vi "Teleop.vi"(0 "Call Context":T10) -> (6 "SubState 3":T4, 8 "SubState 4":T4, 9 "SubState 5":T9, 11 "Loop 3 Data":T5, 13 "Loop 4 Data":T3, 14 "SubState 0":T4=enum."driver control", 15 "Loop 1 Data":T7, 16 "Loop 0 Data":T8, 17 "SubState 1":T4, 18 "Loop 2 Data":T6, 19 "SubState 2":T4)   [LabVIEW 2013]
uses:
  typedefs/subStates.ctl
  <vilib>/Rock Robotics/WPI/DriverStation/WPI_DriverStationDerivedRobotMode.ctl
  typedefs/singleUseSubstate.ctl
  typedefs/Loop Datatypes/Loop 0 Datatype.ctl
  typedefs/Loop Datatypes/Loop 1 Datatype.ctl
  typedefs/Loop Datatypes/Loop 2 Datatype.ctl
  typedefs/Loop Datatypes/Loop 3 Datatype.ctl
  typedefs/Loop Datatypes/Loop 4 Datatype.ctl
  <vilib>/Rock Robotics/WPI/Joystick/WPI_JoystickDevRef.ctl
  <vilib>/Rock Robotics/WPI/Joystick/WPI_JoystickDeviceEnum.ctl
  typedefs/fg_typedef.ctl
  typedefs/vision enable.ctl
  <vilib>/Rock Robotics/WPI/Joystick/WPI_JoystickGetSetRefNum.vi
panel:
  out "JS3":T1
  out "Drive to DC":bool
  out "JS1":T1
  out "JS2":T1
  out "Exit Value":i32=-1
  # "Loop Data and Substates"
  # "Drive Loop"
  # "Shooter Pneumatics Loop"
  # "Pickup/Passing Belts Loop"
  # "Pickup Arm Loop"
  # "Shifter Loop"
  # "Latch Loop"
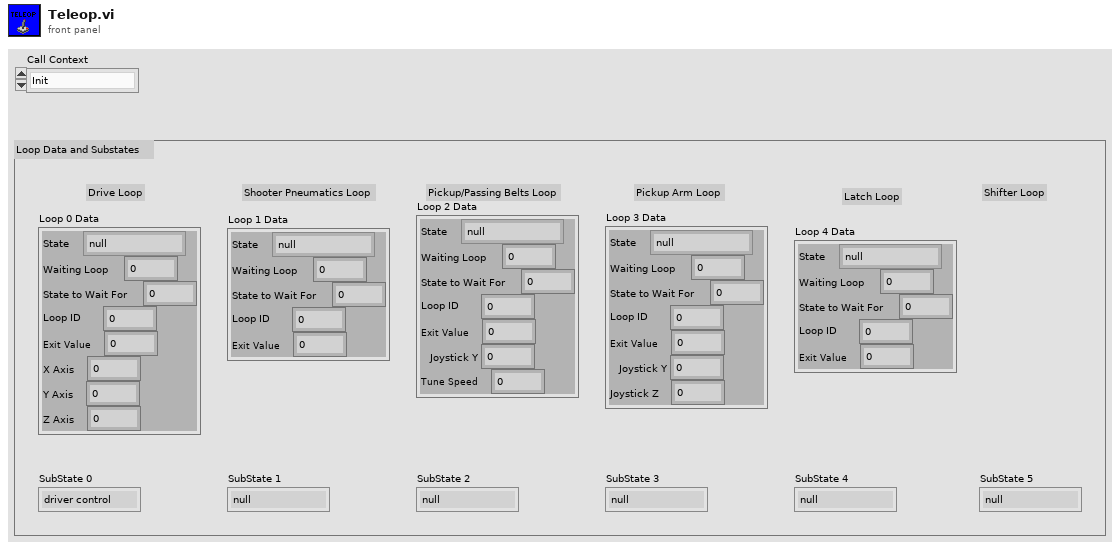
[diagram p1: front panel]
types:
  T1 = typedef "WPI_JoystickDevRef.ctl" = cluster{"Device":T2}
  T2 = typedef "WPI_JoystickDeviceEnum.ctl" = enum16{"USB 1", "USB 2", "USB 3", "USB 4", "Kinect 1", "Kinect 2"}
  T3 = typedef "Loop 4 Datatype.ctl" = cluster{"State":T4, "Waiting Loop":i32, "State to Wait For":i32, "Loop ID":i32, "Exit Value":i32}
  T4 = typedef "subStates.ctl" = enum16{"null", "wait", "driver control", "auto", "manual override", "hold position", "rotate", "pickup", "pass", "load", "goto shoot", "shoot", "end"}
  T5 = typedef "Loop 3 Datatype.ctl" = cluster{"State":T4, "Waiting Loop":i32, "State to Wait For":i32, "Loop ID":i32, "Exit Value":i32, "Joystick Y":dbl, "Joystick Z":dbl}
  T6 = typedef "Loop 2 Datatype.ctl" = cluster{"State":T4, "Waiting Loop":i32, "State to Wait For":i32, "Loop ID":i32, "Exit Value":i32, "Joystick Y":dbl, "Tune Speed":dbl}
  T7 = typedef "Loop 1 Datatype.ctl" = cluster{"State":T4, "Waiting Loop":i32, "State to Wait For":i32, "Loop ID":i32, "Exit Value":i32}
  T8 = typedef "Loop 0 Datatype.ctl" = cluster{"State":T4, "Waiting Loop":i32, "State to Wait For":i32, "Loop ID":i32, "Exit Value":i32, "X Axis":dbl, "Y Axis":dbl, "Z Axis":dbl}
  T9 = typedef "singleUseSubstate.ctl" = enum16{"null", "wait", "shift high", "shift low"}
  T10 = typedef "WPI_DriverStationDerivedRobotMode.ctl" = enum16{"Init", "Execute", "Stop"}
  T11 = cluster{"axis 1 (x)":dbl, "axis 2 (y)":dbl, "axis 3 (throttle)":dbl, "axis 4":dbl, "axis 5":dbl, "axis 6":dbl}
  T12 = typedef "WPI_EncoderDevRef.ctl" = cluster{"DevStatus":errorcluster, "EncoderIndex":T13, "CounterIndex":T14, "DistancePerCount":dbl, "Decoding Type":T15}
  T13 = typedef "FPGA_EncoderIdx.ctl" = enum8{"Enc 0", "Enc 1", "Enc 2", "Enc 3", "Invalid"}
  T14 = typedef "FPGA_CounterCtrSystemIndex.ctl" = enum8{"Ctr 0", "Ctr 1", "Ctr 2", "Ctr 3", "Ctr 4", "Ctr 5", "Ctr 6", "Ctr 7", "Invalid"}
  T15 = typedef "WPI_EncoderType.ctl" = enum16{"1x", "2x", "4x"}
  T16 = typedef "vision enable.ctl" = enum16{"Enable", "Disable", "Stop"}
  T17 = typedef "fg_typedef.ctl" = enum16{"Get", "Set"}
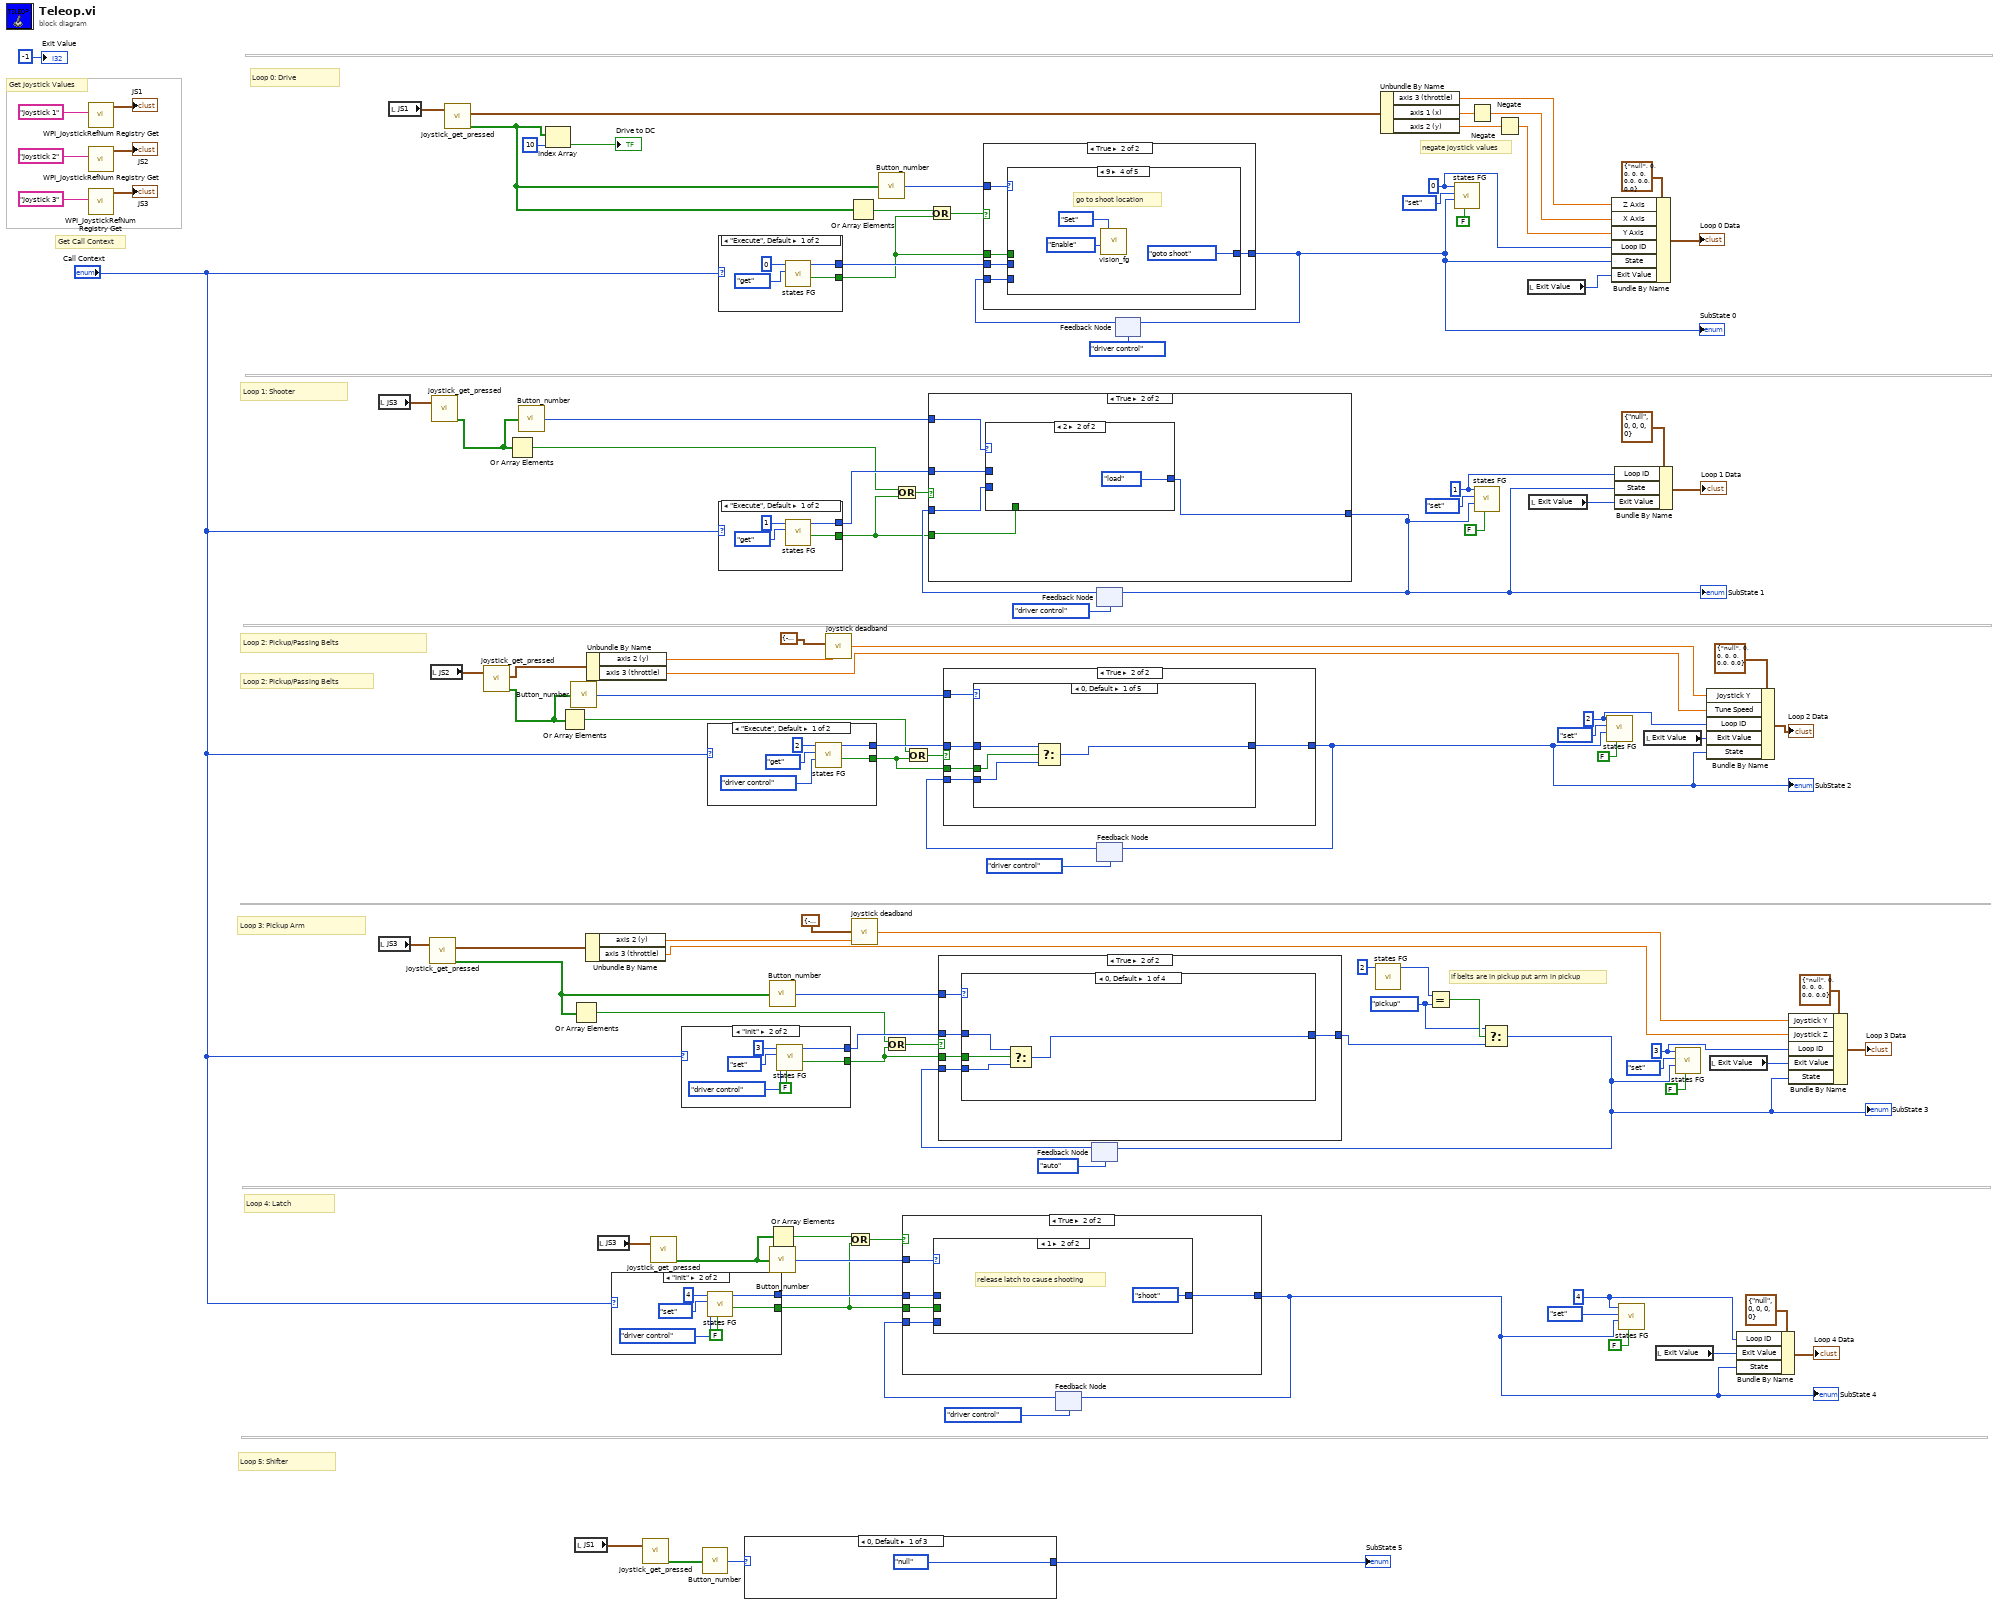
[diagram p0: block diagram]
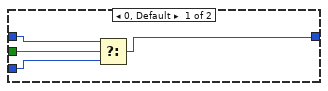
[diagram p3: hidden frame]
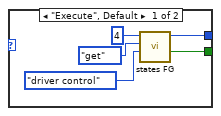
[diagram p4: hidden frame]
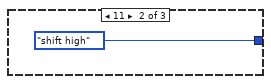
[diagram p5: hidden frame]
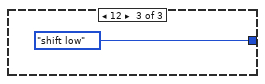
[diagram p6: hidden frame]
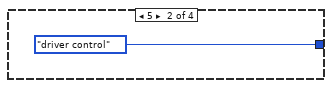
[diagram p8: hidden frame]
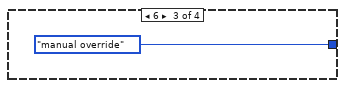
[diagram p9: hidden frame]
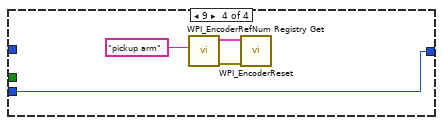
[diagram p10: hidden frame]
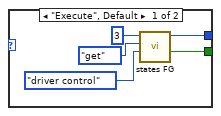
[diagram p11: hidden frame]
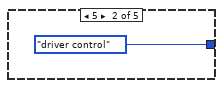
[diagram p13: hidden frame]
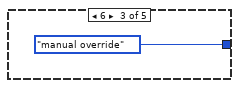
[diagram p14: hidden frame]
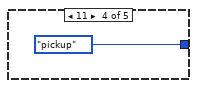
[diagram p15: hidden frame]
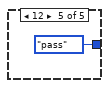
[diagram p16: hidden frame]
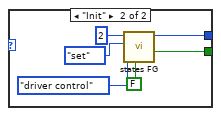
[diagram p17: hidden frame]
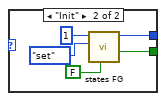
[diagram p18: hidden frame]
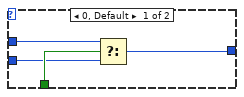
[diagram p20: hidden frame]
diagram:
  w1 = subStates."pickup" ("y")
  w20 = 4 ("Loop ID")
  w87 = 3 ("Loop ID")
  w88 = 2 ("Loop ID")
  w97 = 1 ("Loop ID")
  w99 = 0 ("Loop ID")
  # "if belts are in pickup put arm in pickup"
  # "Loop 2: Pickup/Passing Belts"
  # "negate joystick values"
  # "Get Call Context"
  # "Get Joystick Values"
  # "Loop 4: Latch"
  # "Loop 3: Pickup Arm"
  # "Loop 5: Shifter"
  # "Loop 2: Pickup/Passing Belts"
  # "Loop 1: Shooter"
  # "Loop 0: Drive"
  n1 = call <vilib>:"WPI_JoystickRefNum Registry Get.vi"("refnum name"="Joystick 1") -> ("JoystickDevRef"=→"JS1":T1)  [unwired: 9 in, 1 out]
  n2 = call <vilib>:"WPI_JoystickRefNum Registry Get.vi"("refnum name"="Joystick 2") -> ("JoystickDevRef"=→"JS2":T1)  [unwired: 9 in, 1 out]
  n3 = call <vilib>:"WPI_JoystickRefNum Registry Get.vi"("refnum name"="Joystick 3") -> ("JoystickDevRef"=→"JS3":T1)  [unwired: 9 in, 1 out]
  n4 = local read "JS3"() -> (w64:T1)
  n5 = local read "JS3"() -> (w49:T1)
  n6 = local read "JS1"() -> (w65:T1)
  n7 = call "joystick_get_pressed.vi"("JoystickDevRef 2"=w49) -> ("Axes"=w53:T11, "Buttons Pressed?"=w29:bool[])  [unwired: 1 in, 2 out]
  n8 = local read "JS2"() -> (w36:T1)
  n9 = call "joystick_get_pressed.vi"("JoystickDevRef 2"=w64) -> ("Buttons Pressed?"=w31:bool[])  [unwired: 1 in, 3 out]
  n10 = call "joystick_get_pressed.vi"("JoystickDevRef 2"=w65) -> ("Axes"=w69:T11, "Buttons Pressed?"=w44:bool[])  [unwired: 1 in, 2 out]
  n11 = call "joystick_get_pressed.vi"("JoystickDevRef 2"=w36) -> ("Axes"=w17:T11, "Buttons Pressed?"=w18:bool[])  [unwired: 1 in, 2 out]
  n12 = Or Array Elements(Boolean array=w31) -> (logical OR=w56:bool)
  n13 = call "Button_number.vi"("Button Array"=w31) -> ("Button Pressed"=w58:i32)
  n14 = Index Array(array=w44, index=10) -> (element=→"Drive to DC":bool)
  n15 = Or Array Elements(Boolean array=w18) -> (logical OR=w35:bool)
  n16 = call "Button_number.vi"("Button Array"=w18) -> ("Button Pressed"=w34:i32)
  n17 = Or Array Elements(Boolean array=w29) -> (logical OR=w52:bool)
  n18 = local read "JS1"() -> (w39:T1)
  n19 = Unbundle By Name(w53) -> ("axis 2 (y)"=w47:dbl, "axis 3 (throttle)"=w13:dbl)
  n20 = Unbundle By Name(w17) -> ("axis 2 (y)"=w28:dbl, "axis 3 (throttle)"=w15:dbl)
  n21 = local read "JS3"() -> (w12:T1)
  n22 = case shown="\"Init\"" "Call Context" {
    tunnel: [w118 w124] -> w7
    tunnel: [w116 w121] -> w22
    frame "Execute", Default {
      n23 = call "states FG.vi"("subState in"=subStates."driver control", "menu (get)"=enum16{"set", "get"}."get", "Loop ID"=4) -> ("exit out"=w118:bool, "subState out"=w116:T4)  [unwired: 5 in, 2 out]
    }
    frame "Init" {
      n24 = call "states FG.vi"("exit in"=FALSE, "subState in"=subStates."driver control", "menu (get)"=enum16{"set", "get"}."set", "Loop ID"=4) -> ("exit out"=w124:bool, "subState out"=w121:T4)  [unwired: 4 in, 2 out]
    }
  }
  n25 = call "joystick_get_pressed.vi"("JoystickDevRef 2"=w39) -> ("Buttons Pressed?"=w41:bool[])  [unwired: 1 in, 3 out]
  n26 = call "joystick_get_pressed.vi"("JoystickDevRef 2"=w12) -> ("Buttons Pressed?"=w11:bool[])  [unwired: 1 in, 3 out]
  n27 = case shown="\"Init\"" "Call Context" {
    tunnel: [w129 w135] -> w50
    tunnel: [w127 w132] -> w85
    frame "Execute", Default {
      n28 = call "states FG.vi"("subState in"=subStates."driver control", "menu (get)"=enum16{"set", "get"}."get", "Loop ID"=3) -> ("exit out"=w129:bool, "subState out"=w127:T4)  [unwired: 5 in, 2 out]
    }
    frame "Init" {
      n29 = call "states FG.vi"("exit in"=FALSE, "subState in"=subStates."driver control", "menu (get)"=enum16{"set", "get"}."set", "Loop ID"=3) -> ("exit out"=w135:bool, "subState out"=w132:T4)  [unwired: 4 in, 2 out]
    }
  }
  n30 = call "Button_number.vi"("Button Array"=w41) -> ("Button Pressed"=w40:i32)
  n31 = case shown="\"Execute\", Default" "Call Context" {
    tunnel: [w140 w146] -> w55
    tunnel: [w138 w143] -> w104
    frame "Execute", Default {
      n32 = call "states FG.vi"("subState in"=subStates."driver control", "menu (get)"=enum16{"set", "get"}."get", "Loop ID"=2) -> ("exit out"=w140:bool, "subState out"=w138:T4)  [unwired: 5 in, 2 out]
    }
    frame "Init" {
      n33 = call "states FG.vi"("exit in"=FALSE, "subState in"=subStates."driver control", "menu (get)"=enum16{"set", "get"}."set", "Loop ID"=2) -> ("exit out"=w146:bool, "subState out"=w143:T4)  [unwired: 4 in, 2 out]
    }
  }
  n34 = case shown="\"Execute\", Default" "Call Context" {
    tunnel: [w150 w155] -> w62
    tunnel: [w149 w153] -> w102
    frame "Execute", Default {
      n35 = call "states FG.vi"("menu (get)"=enum16{"set", "get"}."get", "Loop ID"=0) -> ("exit out"=w150:bool, "subState out"=w149:T4)  [unwired: 6 in, 2 out]
    }
    frame "Init" {
      n36 = call "states FG.vi"("exit in"=FALSE, "menu (get)"=enum16{"set", "get"}."set", "Loop ID"=0) -> ("exit out"=w155:bool, "subState out"=w153:T4)  [unwired: 5 in, 2 out]
    }
  }
  n37 = case shown="\"Execute\", Default" "Call Context" {
    tunnel: [w159 w164] -> w59
    tunnel: [w158 w162] -> w101
    frame "Execute", Default {
      n38 = call "states FG.vi"("menu (get)"=enum16{"set", "get"}."get", "Loop ID"=1) -> ("exit out"=w159:bool, "subState out"=w158:T4)  [unwired: 6 in, 2 out]
    }
    frame "Init" {
      n39 = call "states FG.vi"("exit in"=FALSE, "menu (get)"=enum16{"set", "get"}."set", "Loop ID"=1) -> ("exit out"=w164:bool, "subState out"=w162:T4)  [unwired: 5 in, 2 out]
    }
  }
  n40 = case shown="0, Default" w40 {
    tunnel: [singleUseSubstate."null" ("Enum") singleUseSubstate."shift high" ("Enum") singleUseSubstate."shift low" ("Enum")] -> w77
    frame 0, Default {
    }
    frame 11 {
    }
    frame 12 {
    }
  }
  "SubState 5" <- w77
  n41 = call "Button_number.vi"("Button Array"=w29) -> ("Button Pressed"=w51:i32)
  n42 = call "Button_number.vi"("Button Array"=w11) -> ("Button Pressed"=w8:i32)
  n43 = Or Array Elements(Boolean array=w11) -> (logical OR=w10:bool)
  n44 = call "joystick deadband.vi"("Joystick In"=w28, "Deadband Range"=cluster{"Deadband Min":dbl, "Deadband Max":dbl} {"Deadband Min"=-0.05, "Deadband Max"=0.05}) -> ("Joystick Out"=w16:dbl)  [unwired: 4 in]
  n45 = Or(x=w10, y=w7) -> (x .or. y?=w9:bool)
  n46 = Or Array Elements(Boolean array=w44) -> (logical OR=w63:bool)
  n47 = call "joystick deadband.vi"("Joystick In"=w47, "Deadband Range"=cluster{"Deadband Min":dbl, "Deadband Max":dbl} {"Deadband Min"=-0.05, "Deadband Max"=0.05}) -> ("Joystick Out"=w14:dbl)  [unwired: 4 in]
  n48 = call "Button_number.vi"("Button Array"=w44) -> ("Button Pressed"=w68:i32)
  n49 = Or(x=w52, y=w50) -> (x .or. y?=w54:bool)
  n50 = Or(x=w56, y=w59) -> (x .or. y?=w60:bool)
  n51 = Or(x=w35, y=w55) -> (x .or. y?=w57:bool)
  n52 = Or(x=w63, y=w62) -> (x .or. y?=w61:bool)
  n53 = feedback #1(subStates."driver control" ("Drive SubState")) -> (w25:T4)
  n54 = case shown="True" w9 {
    tunnel: w25 -> [w170 w172]
    tunnel: [w170 w171] -> w48
    tunnel: w22 -> [_ w174]
    tunnel: w8 -> [_ w175]
    tunnel: w7 -> [_ w173]
    frame False {
      # "*yawn* nothing to do...wire through the previous state"
    }
    frame True {
      n55 = case shown="1" w175 {
        tunnel: w174 -> [w178 _]
        tunnel: w173 -> [w179 _]
        tunnel: w172 -> [w177 _]
        tunnel: [w176 subStates."shoot" ("Drive SubState")] -> w171
        frame 0, Default {
          n56 = Select(t=w178, s=w179, f=w177) -> (s? t:f=w176:T4)
        }
        frame 1 {
          # "release latch to cause shooting"
        }
      }
    }
  }
  "SubState 4" <- w48
  n57 = feedback-in #1(w48) -> ()
  n58 = feedback #2(subStates."auto" ("Drive SubState")) -> (w82:T4)
  n59 = case shown="True" w54 {
    tunnel: w82 -> [w181 w182]
    tunnel: [w181 w183] -> w4
    tunnel: w85 -> [_ w184]
    tunnel: w51 -> [_ w186]
    tunnel: w50 -> [_ w185]
    frame False {
      # "boring drivers, not pressing anything...wire through the previous state"
    }
    frame True {
      n60 = case shown="0, Default" w186 {
        tunnel: w185 -> [w190 _ _ _]
        tunnel: w182 -> [w189 _ _ w196]
        tunnel: w184 -> [w188 _ _ _]
        tunnel: [w187 subStates."driver control" ("Drive SubState") subStates."manual override" ("Drive SubState") w196] -> w183
        frame 0, Default {
          n61 = Select(t=w188, s=w190, f=w189) -> (s? t:f=w187:T4)
        }
        frame 5 {
        }
        frame 6 {
        }
        frame 9 {
          n62 = call <vilib>:"WPI_EncoderRefNum Registry Get.vi"("refnum name"="pickup arm") -> ("error out"=w194:errorcluster, "EncoderDevRef"=w193:T12)  [unwired: 9 in]
          n63 = call <vilib>:"WPI_EncoderReset.vi"("error in (no error)"=w194, "EncoderDevRef"=w193) -> ()  [unwired: 8 in, 2 out]
        }
      }
    }
  }
  n64 = feedback #3(subStates."driver control" ("Drive SubState")) -> (w103:T4)
  n65 = case shown="True" w60 {
    tunnel: w103 -> [w197 w201]
    tunnel: [w197 w198] -> w70
    tunnel: w101 -> [_ w202]
    tunnel: w58 -> [_ w200]
    tunnel: w59 -> [_ w199]
    frame False {
      # "nothing pressed here, move along (wire through the previous state)"
    }
    frame True {
      n66 = case shown="2" w200 {
        tunnel: w202 -> [w205 _]
        tunnel: w201 -> [w204 _]
        tunnel: [w203 subStates."load" ("Drive SubState")] -> w198
        tunnel: w199 -> [w206 _]
        frame 0, Default {
          n67 = Select(t=w205, s=w206, f=w204) -> (s? t:f=w203:T4)
        }
        frame 2 {
        }
      }
    }
  }
  "SubState 1" <- w70
  n68 = feedback-in #3(w70) -> ()
  n69 = feedback #4(subStates."driver control" ("Drive SubState")) -> (w107:T4)
  n70 = case shown="True" w57 {
    tunnel: w107 -> [w208 w210]
    tunnel: [w208 w209] -> w27
    tunnel: w104 -> [_ w211]
    tunnel: w34 -> [_ w213]
    tunnel: w55 -> [_ w212]
    frame False {
      # "nothing pressed here, move along obviously and wire through the previous state"
    }
    frame True {
      n71 = case shown="0, Default" w213 {
        tunnel: w212 -> [w217 _ _ _ _]
        tunnel: w211 -> [w216 _ _ _ _]
        tunnel: w210 -> [w215 _ _ _ _]
        tunnel: [w214 subStates."driver control" ("Drive SubState") subStates."manual override" ("Drive SubState") subStates."pickup" ("Drive SubState") subStates."pass" ("Drive SubState")] -> w209
        frame 0, Default {
          n72 = Select(t=w216, s=w217, f=w215) -> (s? t:f=w214:T4)
        }
        frame 5 {
        }
        frame 6 {
        }
        frame 11 {
        }
        frame 12 {
        }
      }
    }
  }
  "SubState 2" <- w27
  n73 = feedback-in #4(w27) -> ()
  n74 = feedback #5(subStates."driver control" ("Drive SubState")) -> (w109:T4)
  n75 = case shown="True" w61 {
    tunnel: w109 -> [w222 w224]
    tunnel: [w222 w223] -> w38
    tunnel: w102 -> [_ w225]
    tunnel: w68 -> [_ w227]
    tunnel: w62 -> [_ w226]
    frame False {
      # "keep current state, no change necessary"
    }
    frame True {
      n76 = case shown="9" w227 {
        tunnel: w226 -> [w231 _ _ _ _]
        tunnel: w225 -> [w230 _ _ _ _]
        tunnel: w224 -> [w229 _ w235 _ w250]
        tunnel: [w228 subStates."driver control" ("Drive SubState") w235 subStates."goto shoot" ("Drive SubState") w246] -> w223
        frame 0, Default {
          n77 = Select(t=w230, s=w231, f=w229) -> (s? t:f=w228:T4)
        }
        frame 7 {
          # "put robot drive in driver control"
          n78 = call "vision_fg.vi"("Action"=vision_enable."Disable", "Menu"=fg_typedef."Set") -> ()  [unwired: 1 in, 2 out]
        }
        frame 8 {
          w238 = vision_enable."Enable" ("y")
          # "toggle vision"
          n79 = call "vision_fg.vi"("Menu"=fg_typedef."Get") -> ("State Out"=w240:T16)  [unwired: 2 in, 1 out]
          n80 = Equal?(x=w240, y=w238) -> (x = y?=w239:bool)
          n81 = Select(t=vision_enable."Disable" ("y"), s=w239, f=w238) -> (s? t:f=w236:T16)
          n82 = call "vision_fg.vi"("Action"=w236, "Menu"=fg_typedef."Set") -> ()  [unwired: 1 in, 2 out]
        }
        frame 9 {
          # "go to shoot location"
          n83 = call "vision_fg.vi"("Action"=vision_enable."Enable", "Menu"=fg_typedef."Set") -> ()  [unwired: 1 in, 2 out]
        }
        frame 10 {
          w247 = subStates."hold position" ("x")
          # "button 10, hold position toggle"
          n84 = Equal?(x=w247, y=w250) -> (x = y?=w249:bool)
          n85 = Select(t=subStates."driver control" ("Drive SubState"), s=w249, f=w247) -> (s? t:f=w246:T4)
        }
      }
    }
  }
  "SubState 0" <- w38
  n86 = feedback-in #5(w38) -> ()
  n87 = call "states FG.vi"("Loop ID"=2) -> ("subState out"=w5:T4)  [unwired: 7 in, 3 out]
  n88 = Unbundle By Name(w69) -> ("axis 3 (throttle)"=w45:dbl, "axis 1 (x)"=w74:dbl, "axis 2 (y)"=w73:dbl)
  n89 = Equal?(x=w5, y=w1) -> (x = y?=w2:bool)
  n90 = call "states FG.vi"("exit in"=FALSE, "subState in"=w38, "menu (get)"=enum16{"set", "get"}."set", "Loop ID"=w99) -> ()  [unwired: 4 in, 4 out]
  n91 = Negate(x=w74) -> (-x=w72:dbl)
  n92 = call "states FG.vi"("exit in"=FALSE, "subState in"=w70, "menu (get)"=enum16{"set", "get"}."set", "Loop ID"=w97) -> ()  [unwired: 4 in, 4 out]
  n93 = Select(t=w1, s=w2, f=w4) -> (s? t:f=w3:T4)
  "SubState 3" <- w3
  n94 = feedback-in #2(w3) -> ()
  n95 = Negate(x=w73) -> (-x=w71:dbl)
  n96 = local read "Exit Value"() -> (w95:i32)
  n97 = local read "Exit Value"() -> (w94:i32)
  n98 = call "states FG.vi"("exit in"=FALSE, "subState in"=w27, "menu (get)"=enum16{"set", "get"}."set", "Loop ID"=w88) -> ()  [unwired: 4 in, 4 out]
  n99 = Bundle By Name(cluster=T8 {"State"=enum."null", "Waiting Loop"=0, "State to Wait For"=0, "Loop ID"=0, "Exit Value"=0, "X Axis"=0.0, "Y Axis"=0.0, "Z Axis"=0.0} ("Cluster"), "Z Axis"=w45, "X Axis"=w72, "Y Axis"=w71, "Loop ID"=w99, "State"=w38, "Exit Value"=w95) -> (→"Loop 0 Data":T8)
  n100 = Bundle By Name(cluster=T7 {"State"=enum."null", "Waiting Loop"=0, "State to Wait For"=0, "Loop ID"=0, "Exit Value"=0} ("Cluster"), "Loop ID"=w97, "State"=w70, "Exit Value"=w94) -> (→"Loop 1 Data":T7)
  n101 = call "states FG.vi"("exit in"=FALSE, "subState in"=w48, "menu (get)"=enum16{"set", "get"}."set", "Loop ID"=w20) -> ()  [unwired: 4 in, 4 out]
  n102 = local read "Exit Value"() -> (w89:i32)
  n103 = local read "Exit Value"() -> (w21:i32)
  n104 = call "states FG.vi"("exit in"=FALSE, "subState in"=w3, "menu (get)"=enum16{"set", "get"}."set", "Loop ID"=w87) -> ()  [unwired: 4 in, 4 out]
  n105 = Bundle By Name(cluster=T6 {"State"=enum."null", "Waiting Loop"=0, "State to Wait For"=0, "Loop ID"=0, "Exit Value"=0, "Joystick Y"=0.0, "Tune Speed"=0.0} ("Loop 2 Data"), "Joystick Y"=w16, "Tune Speed"=w15, "Loop ID"=w88, "Exit Value"=w89, "State"=w27) -> (→"Loop 2 Data":T6)
  n106 = local read "Exit Value"() -> (w86:i32)
  n107 = Bundle By Name(cluster=T3 {"State"=enum."null", "Waiting Loop"=0, "State to Wait For"=0, "Loop ID"=0, "Exit Value"=0} ("Loop 4 Data"), "Loop ID"=w20, "Exit Value"=w21, "State"=w48) -> (→"Loop 4 Data":T3)
  n108 = Bundle By Name(cluster=T5 {"State"=enum."null", "Waiting Loop"=0, "State to Wait For"=0, "Loop ID"=0, "Exit Value"=0, "Joystick Y"=0.0, "Joystick Z"=0.0} ("Loop 3 Data"), "Joystick Y"=w14, "Joystick Z"=w13, "Loop ID"=w87, "Exit Value"=w86, "State"=w3) -> (→"Loop 3 Data":T5)
  "Exit Value" <- -1 ("Exit Value")
